vi "Shooter Controller.vi"(8 "error in":errorcluster) -> ()   [LabVIEW 2019]
doc: "This VI executes continuously carrying out the current operation and responding to updates or new operations. It will often contain the timing or control code that is difficult to place directly in TeleOp. This VI generally opens all sensors and motors and isolates the rest of the robot code from knowing how the operations are carried out."
uses:
  <vilib>/Rock Robotics/WPI/Framework/Completion Status.ctl
  Shooter Setpoints.ctl
  Shooter Operations.ctl
  <vilib>/Rock Robotics/WPI/ThirdParty/REV Robotics/SPARK MAX/Typedef/Spark MAX Idle Mode.ctl
  <vilib>/Rock Robotics/WPI/ThirdParty/REV Robotics/SPARK MAX/Typedef/Spark MAX Control Type.ctl
  <vilib>/Rock Robotics/Network Tables/NT Read Boolean.vi
  Framework/Robot Global Data.vi
  <vilib>/Rock Robotics/Network Tables/NT Read Number.vi
  <vilib>/Rock Robotics/Network Tables/NT Write Number.vi
  <vilib>/Rock Robotics/Network Tables/NT Write Boolean.vi
panel:
  out "Waveform Chart 2":dbl(graph)
  out "Waveform Chart":dbl(graph)
  in  "Interactive Values":T1
  out "Current\nCmd":string
  in  "Buttons":cluster{"Execute Cmd":bool, "Abort Cmd":bool}
  out "Command Timing":cluster{"Start Time (ms)":u32, "Iterations":i32}
  out "Status":T3
  # "Tip: It may be helpful to observe inputs and sensor values.\nYou may also want to display tuning or debugging controls."
  # "80 amps, old PID"
  # "Interactive Command: You may fill in the settings for a command\nand schedule it with the Execute button. You can observe and abort\nany command while fine tuning the code for the controller."
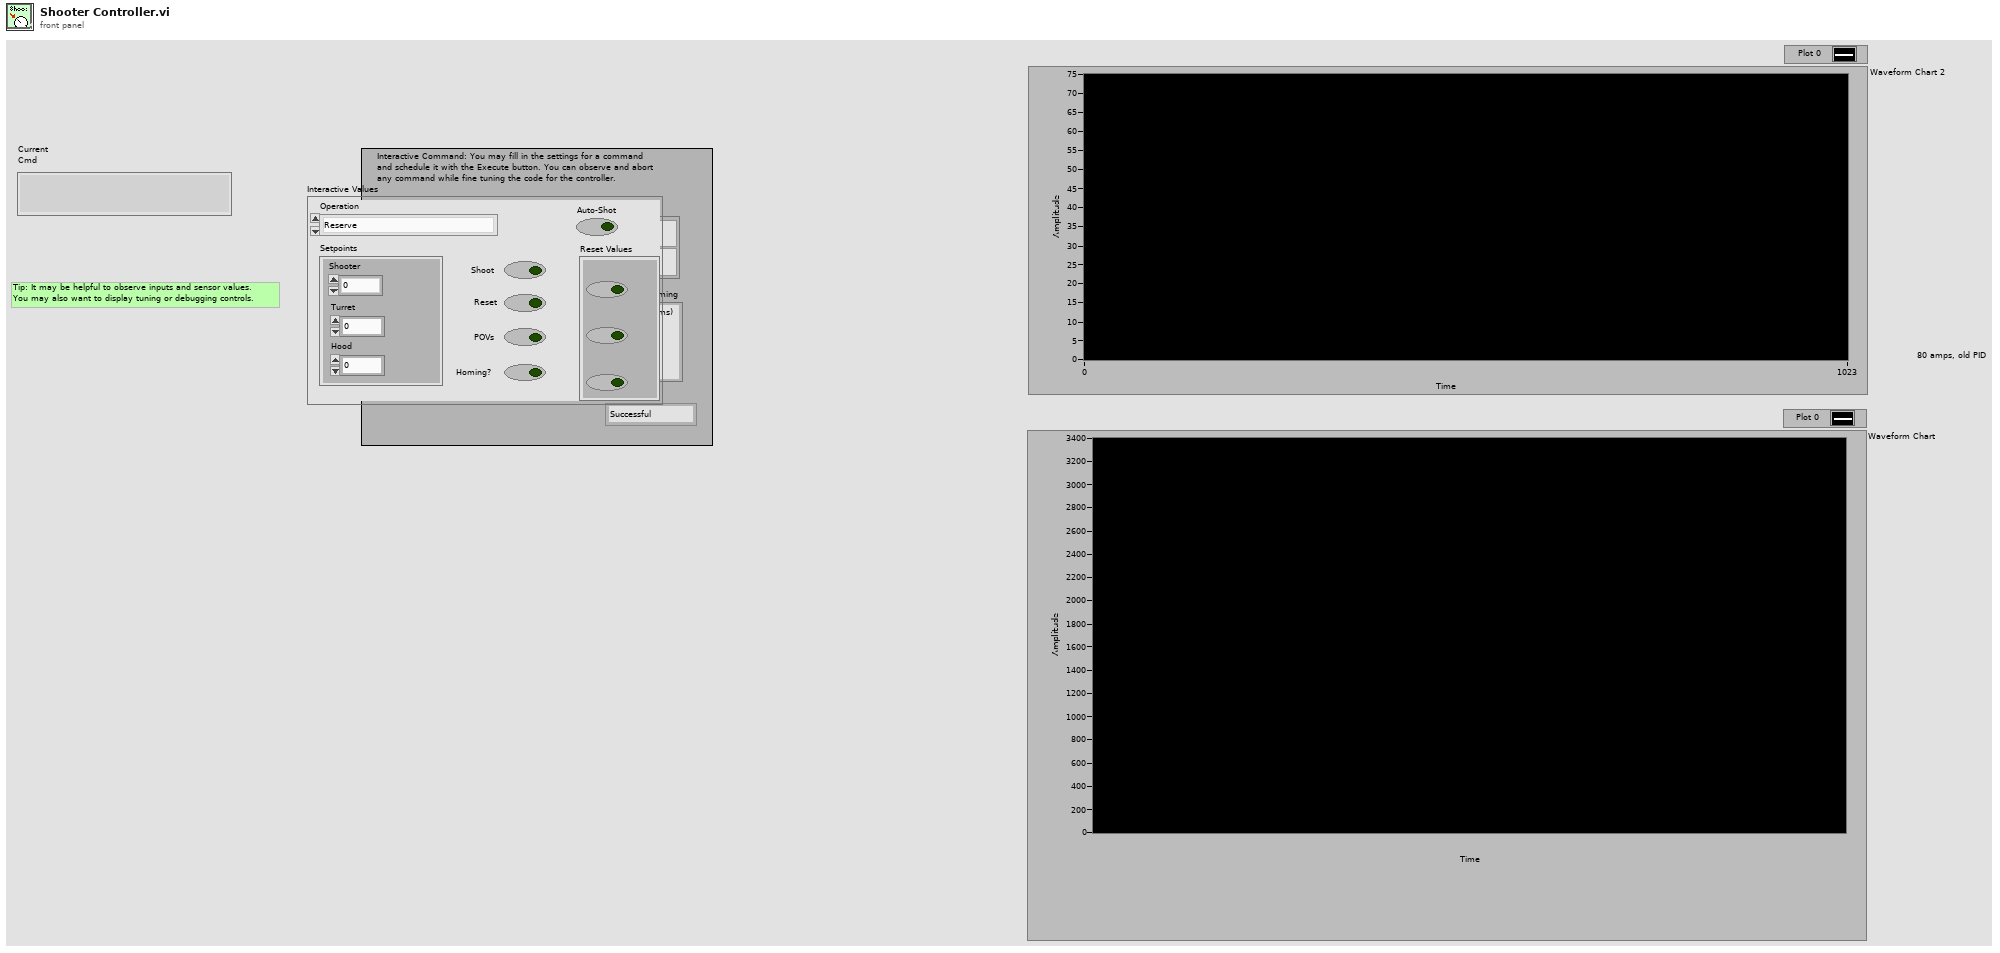
[diagram p1: front panel]
types:
  T1 = typedef "Shooter Setpoints.ctl" = cluster{"Operation":T2, "Setpoints":cluster{"Shooter":dbl, "Turret":dbl, "Hood":dbl}, "Reset Values":cluster{"Shooter Reset":bool, "Turret Reset":bool, "Hood Reset":bool}, "Auto-Shot":bool, "Shoot":bool, "Reset":bool, "POVs":bool, "Homing?":bool}
  T2 = typedef "Shooter Operations.ctl" = enum16{"Reserve", "Read Current", "Immediate"}
  T3 = typedef "Completion Status.ctl" = enum16{"Successful", "Aborted", "Incomplete"}
  T4 = cluster{"P Gain":dbl, "I Gain":dbl, "D Gain":dbl, "F Gain":dbl, "I Zone":dbl, "Min Output":dbl, "Max Output":dbl}
  T5 = typedef "Spark MAX Idle Mode.ctl" = enum16{"Coast", "Brake"}
  T6 = typedef "WPI_MotorControlDeviceRef.ctl" = cluster{"DeviceStatus":errorcluster, "Type":T7, "PWM":cluster{"PWM Channel":T8, "DeadBand":T9}, "CAN":cluster{"Device Number":u8, "SetOutput VI Ref":variant, "GetOutput VI Ref":variant, "Enable VI Ref":variant, "Disable VI Ref":variant, "Data":variant}, "Invert":bool, "DIO PWM":cluster{"PWM \"Enable\" Channel":T8, "DIOChannel":T10, "PWM Rate":dbl}}
  T7 = typedef "WPI_MotorControlType.ctl" = enum16{"PWM", "CAN", "DIO PWM"}
  T8 = typedef "FPGA_DIOPWMChannel.ctl" = enum8{"PWM 0", "PWM 1", "PWM 2", "PWM 3", "PWM 4", "PWM 5", "PWM 6", "PWM 7", "PWM 8", "PWM 9", "PWM MXP 0", "PWM MXP 1", "PWM MXP 2", "PWM MXP 3", "PWM MXP 4", "PWM MXP 5", "PWM MXP 6", "PWM MXP 7", "PWM MXP 8", "PWM MXP 9", "Invalid"}
  T9 = typedef "WPI_PWMDeadband.ctl" = cluster{"Name":string, "maxPositivePwm":i32, "minPositivePwm":i32, "centerPwm":i32, "maxNegativePwm":i32, "minNegativePwm":i32, "angularRange":u16}
  T10 = typedef "FPGA_DIOChannel.ctl" = enum8{"DIO 0", "DIO 1", "DIO 2", "DIO 3", "DIO 4", "DIO 5", "DIO 6", "DIO 7", "DIO 8", "DIO 9", "DIO MXP 0", "DIO MXP 1", "DIO MXP 2", "DIO MXP 3", "DIO MXP 4", "DIO MXP 5", "DIO MXP 6", "DIO MXP 7", "DIO MXP 8", "DIO MXP 9", "DIO MXP 10", "DIO MXP 11", "DIO MXP 12", "DIO MXP 13", "DIO MXP 14", "DIO MXP 15", "SPI Port CS1", "SPI Port CS2", "SPI Port CS3", "SPI Port MISO", "SPI Port MOSI", "Invalid"}
  T11 = typedef "Command Status Info.ctl" = cluster{"Name":string, "Status":T3, "notifier out":T12}
  T12 = typedef "Completion Notifier.ctl" = refnum<notifier>
  T13 = cluster{"Current Command":T1, "Command Timing":cluster{"Start Time (ms)":u32, "Iterations":i32}, "Command Arguments":cluster{"Command Info":T11, "Description":string, "Default Command":T1, "queue out":refnum<queue>, "Subsystem Name":string}}
  T14 = typedef "ADIS16448 Device Reference.ctl" = cluster{"DevStatus":errorcluster, "Hardware Config":T15, "Calibration Complete":refnum<notifier>, "Last Value Reference":refnum<data-value>, "Sychronous Process VI":T18, "Cmd FIFO":refnum<k33>, "Source":T19, "IMU Status LED Pin":T10, "Calibration Time":u32}
  T15 = typedef "ADIS16448 Hardware Configuration.ctl" = cluster{"SPI Clock Rate (Hz)":dbl, "IMU SPI Mode (3)":T16, "IMU Reset Pin":T10, "IMU SPI Bus":T17, "IMU Data Ready Pin":T10, "Stall Config":cluster{"Pow2BytesPerRead":u8, "StallTicks":u16, "CsToSclkTicks":u8}, "IMU Status LED Pin":T10}
  T16 = typedef "WPI_SPIMode.ctl" = enum16{"Mode 0 (Clk Idle Low,Sample on Leading)", "Mode 1 (Clk Idle Low,Sample on Trailing)", "Mode 2 (Clk Idle High,Sample on Leading)", "Mode 3 (Clk Idle High,Sample on Trailing)"}
  T17 = typedef "spi_bus.ctl" = enum16{"SPI On-Board, CS0", "SPI On-Board, CS1", "SPI On-Board, CS2", "SPI On-Board, CS3", "SPI MXP", "Invalid"}
  T18 = typedef "ADIS16448 Process.ctl" = refnum<vi>
  T19 = typedef "FPGA_CounterEncoderSourceConvertionLVSourceType.ctl" = cluster{"DevStatus":errorcluster, "AnalogTriggerMode?":bool, "DigitalMode":cluster{"DIO Channel":T20}, "AnalogTriggerMode":cluster{"AnalogTriggerIndex":T21, "OutputType":T22}}
  T20 = typedef "FPGA_DIODigitalSourceChannel.ctl" = enum8{"DIO 0", "DIO 1", "DIO 2", "DIO 3", "DIO 4", "DIO 5", "DIO 6", "DIO 7", "DIO 8", "DIO 9", "DIO MXP 0", "DIO MXP 1", "DIO MXP 2", "DIO MXP 3", "DIO MXP 4", "DIO MXP 5", "DIO MXP 6", "DIO MXP 7", "DIO MXP 8", "DIO MXP 9", "DIO MXP 10", "DIO MXP 11", "DIO MXP 12", "DIO MXP 13", "DIO MXP 14", "DIO MXP 15", "SPI Port CS1", "SPI Port CS2", "SPI Port CS3", "SPI Port MISO", "SPI Port MOSI", "Disabled"}
  T21 = typedef "FPGA_AnalogTriggerIndex.ctl" = enum8{"Trig 0", "Trig 1", "Trig 2", "Trig 3", "Trig 4", "Trig 5", "Trig 6", "Trig 7", "Invalid"}
  T22 = typedef "FPGA_AnalogTriggerOutType.ctl" = enum16{"InWindow", "TriggerState", "Rising", "Falling"}
  T23 = typedef "Spark MAX Control Type.ctl" = enum16{"Percent VBus", "Voltage", "Velocity", "Position", "Smart Motion", "Current", "Smart Velocity"}
  T24 = cluster{"Shooter Reset":bool, "Turret Reset":bool, "Hood Reset":bool}
  T25 = typedef "ADIS16448 Data.ctl" = cluster{"XAngle":dbl, "YAngle":dbl, "ZAngle":dbl}
  T26 = cluster{u32, "Setpoints":cluster{"Shooter":dbl, "Turret":dbl, "Hood":dbl}}
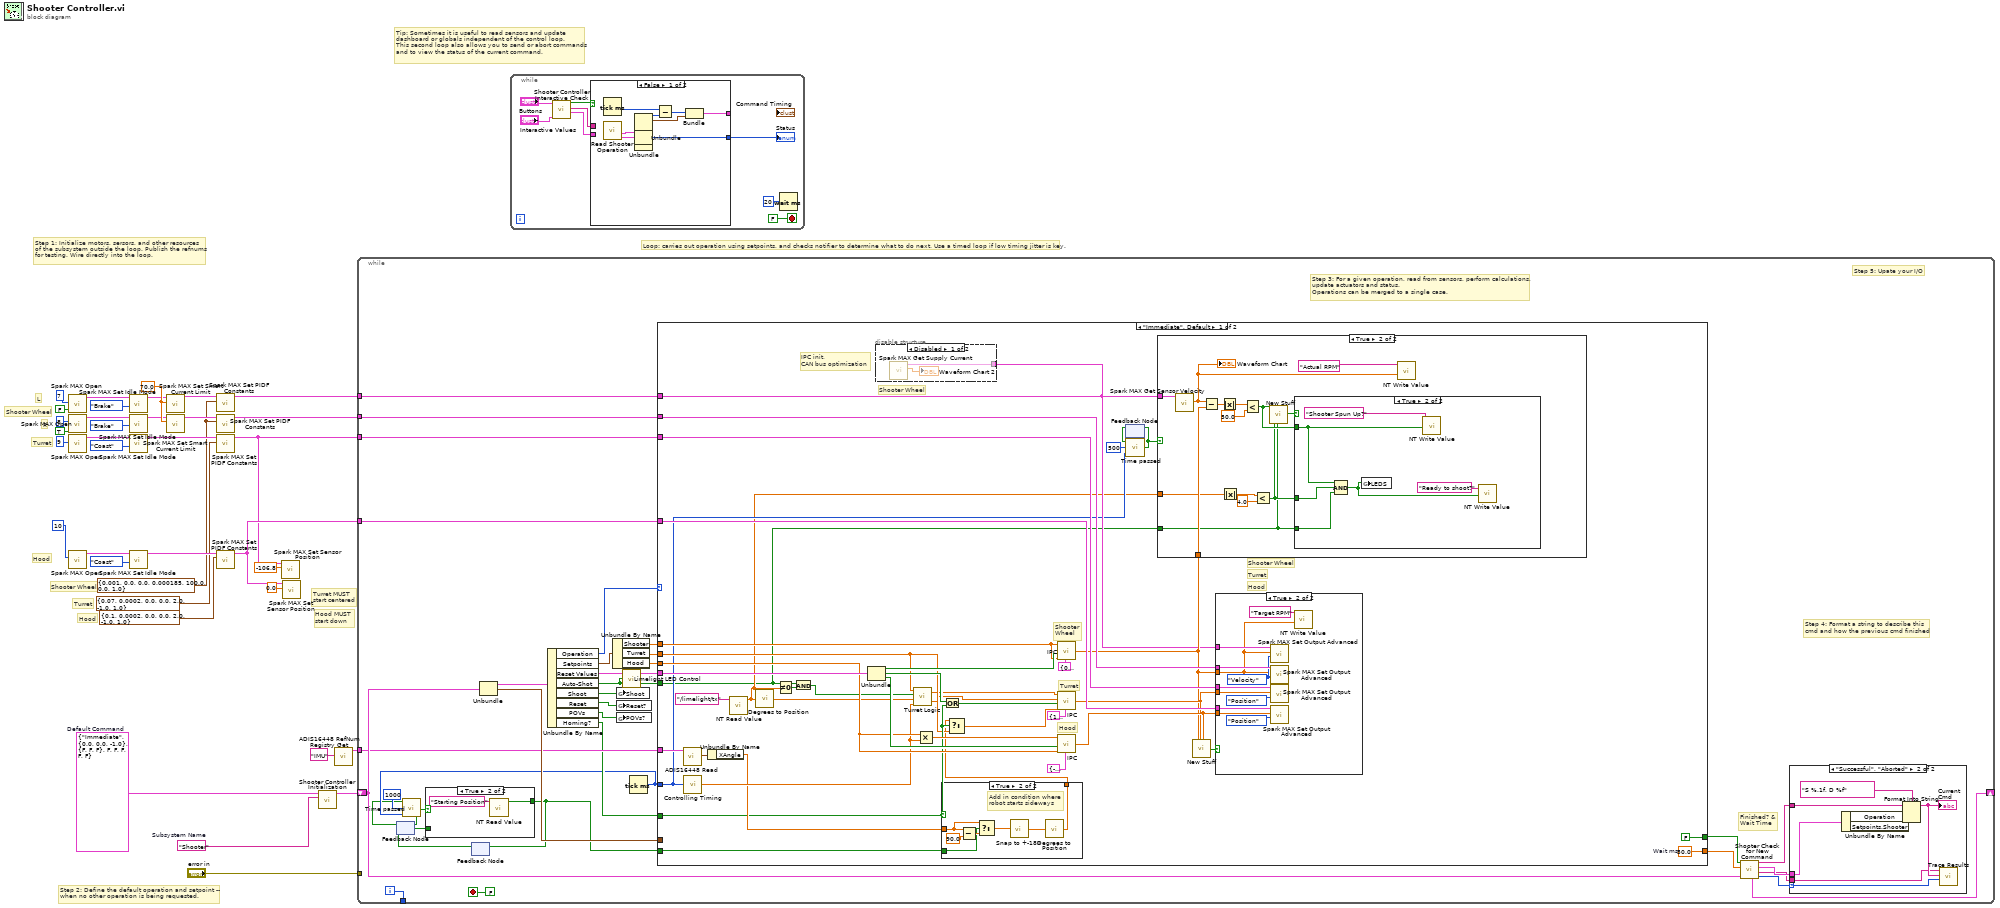
[diagram p0: block diagram]
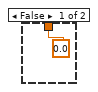
[diagram p6: hidden frame]
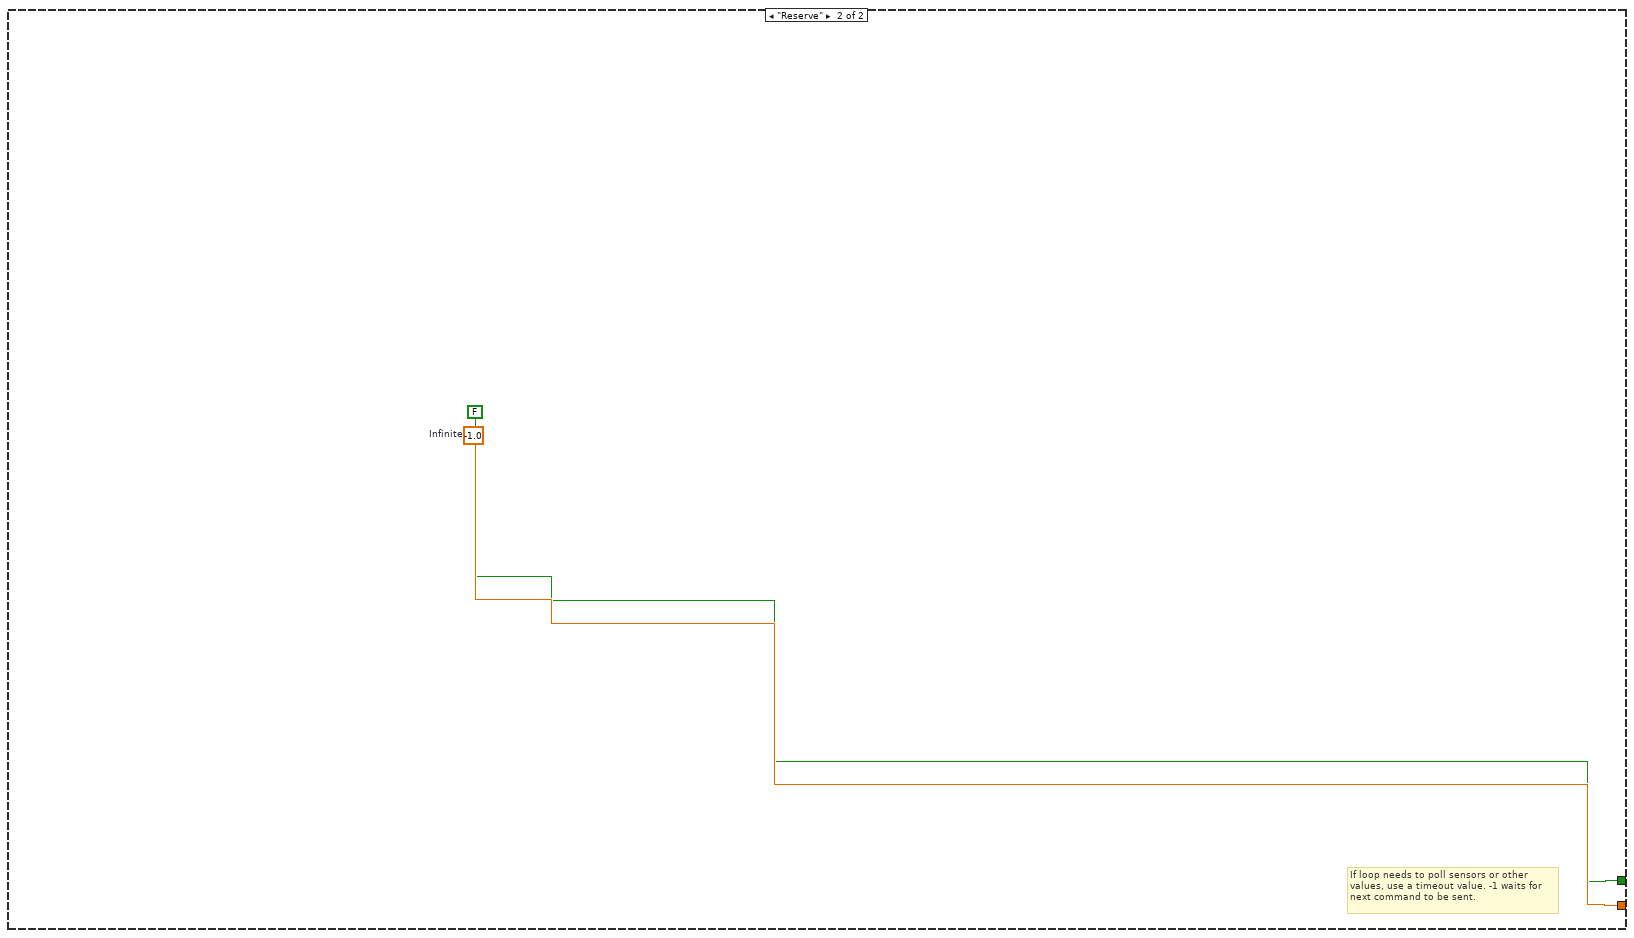
[diagram p8: hidden frame]
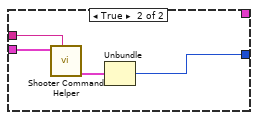
[diagram p10: hidden frame]
diagram:
  w6 = T4 {"P Gain"=0.001, "I Gain"=0.0, "D Gain"=0.0, "F Gain"=0.000185, "I Zone"=100.0, "Min Output"=0.0, "Max Output"=1.0} ("Flywheel PID")
  w26 = 70.0 ("Primay Current Limit (80A)")
  w5 = T1 {"Operation"=enum."Immediate", "Setpoints"={"Shooter"=0.0, "Turret"=0.0, "Hood"=-1.0}, "Reset Values"={"Shooter Reset"=FALSE, "Turret Reset"=FALSE, "Hood Reset"=FALSE}, "Auto-Shot"=FALSE, "Shoot"=FALSE, "Reset"=FALSE, "POVs"=FALSE, "Homing?"=FALSE}  # Default Command
  w34 = "Shooter"  # Subsystem Name
  # "Hood"
  # "Turret"
  # "Shooter Wheel"
  # "R"
  # "L"
  # "Hood MUST\nstart down"
  # "Turret MUST\nstart centered"
  # "Hood"
  # "Turret"
  # "Shooter Wheel"
  # "Tip: Sometimes it is useful to read sensors and update\ndashboard or globals independent of the control loop.\nThis second loop also allows you to send or abort commands\nand to view the status of the current command."
  # "Step 2: Define the default operation and setpoint --\nwhen no other operation is being requested."
  # "Step 1: Initialize motors, sersors, and other resources\nof the subsystem outside the loop. Publish the refnums\nfor testing. Wire directly into the loop."
  # "Loop: carries out operation using setpoints, and checks notifier to determine what to do next. Use a timed loop if low timing jitter is key."
  n1 = call <vilib>:"Spark MAX Open.vi"("Invert"=FALSE, "Device Number"=u8 7) -> ("MotorControlDeviceRef"=w9:T6)  [unwired: 8 in, 1 out]
  n2 = call <vilib>:"Spark MAX Open.vi"("Invert"=TRUE, "Device Number"=u8 8) -> ("MotorControlDeviceRef"=w10:T6)  [unwired: 8 in, 1 out]
  n3 = call <vilib>:"Spark MAX Open.vi"("Device Number"=u8 9) -> ("MotorControlDeviceRef"=w22:T6)  [unwired: 9 in, 1 out]
  n4 = call <vilib>:"Spark MAX Open.vi"("Device Number"=u8 10) -> ("MotorControlDeviceRef"=w21:T6)  [unwired: 9 in, 1 out]
  n5 = call <vilib>:"Spark MAX Set Idle Mode.vi"("Idle Mode"=Spark_MAX_Idle_Mode."Brake", "MotorControlDeviceRef in"=w9) -> ("MotorControlDeviceRef out"=w8:T6)  [unwired: 8 in, 1 out]
  n6 = call <vilib>:"Spark MAX Set Idle Mode.vi"("Idle Mode"=Spark_MAX_Idle_Mode."Brake", "MotorControlDeviceRef in"=w10) -> ("MotorControlDeviceRef out"=w7:T6)  [unwired: 8 in, 1 out]
  n7 = call <vilib>:"Spark MAX Set Idle Mode.vi"("Idle Mode"=Spark_MAX_Idle_Mode."Coast", "MotorControlDeviceRef in"=w22) -> ("MotorControlDeviceRef out"=w20:T6)  [unwired: 8 in, 1 out]
  n8 = call <vilib>:"Spark MAX Set Idle Mode.vi"("Idle Mode"=Spark_MAX_Idle_Mode."Coast", "MotorControlDeviceRef in"=w21) -> ("MotorControlDeviceRef out"=w19:T6)  [unwired: 8 in, 1 out]
  n9 = call <vilib>:"Spark MAX Set Smart Current Limit.vi"("Primay Current Limit (80A)"=w26, "MotorControlDeviceRef in"=w8) -> ("MotorControlDeviceRef out"=w14:T6)  [unwired: 8 in, 1 out]
  n10 = call <vilib>:"Spark MAX Set Smart Current Limit.vi"("Primay Current Limit (80A)"=w26, "MotorControlDeviceRef in"=w7) -> ("MotorControlDeviceRef out"=w15:T6)  [unwired: 8 in, 1 out]
  n11 = call <vilib>:"Spark MAX Set PIDF Constants.vi"("PID Constants"=w6, "MotorControlDeviceRef"=w14) -> ("MotorControlDeviceRef"=w13:T6)  [unwired: 8 in, 1 out]
  n12 = call <vilib>:"Spark MAX Set PIDF Constants.vi"("PID Constants"=w6, "MotorControlDeviceRef"=w15) -> ("MotorControlDeviceRef"=w16:T6)  [unwired: 8 in, 1 out]
  n13 = call <vilib>:"Spark MAX Set PIDF Constants.vi"("PID Constants"=T4 {"P Gain"=0.07, "I Gain"=0.0002, "D Gain"=0.0, "F Gain"=0.0, "I Zone"=2.0, "Min Output"=-1.0, "Max Output"=1.0} ("Turret PID"), "MotorControlDeviceRef"=w20) -> ("MotorControlDeviceRef"=w2:T6)  [unwired: 8 in, 1 out]
  n14 = call <vilib>:"Spark MAX Set PIDF Constants.vi"("PID Constants"=T4 {"P Gain"=0.1, "I Gain"=0.0002, "D Gain"=0.0, "F Gain"=0.0, "I Zone"=2.0, "Min Output"=-1.0, "Max Output"=1.0} ("Hood PID"), "MotorControlDeviceRef"=w19) -> ("MotorControlDeviceRef"=w4:T6)  [unwired: 8 in, 1 out]
  n15 = call <vilib>:"Spark MAX Set Sensor Position.vi"("Position"=-106.8, "MotorControlDeviceRef"=w2) -> ()  [unwired: 8 in, 2 out]
  n16 = call <vilib>:"Spark MAX Set Sensor Position.vi"("Position"=0.0, "MotorControlDeviceRef"=w4) -> ()  [unwired: 8 in, 2 out]
  n17 = call "Shooter Controller Initialization.vi"("Subsystem Name"=w34, "Default Command"=w5) -> ("Current Command"=w35:T13)  [unwired: 9 in]
  n18 = call "ADIS16448 RefNum Registry Get.vi"("refnum name"="IMU") -> ("ADIS16448DevRef Out"=w28:T14)  [unwired: 9 in, 1 out]
  n19 = while {
    shift-right: [w66] -> _
    shift-left: w35 -> [w59]
    tunnel: [w69] -> _
    tunnel: "error in" -> [_]
    tunnel: w16 -> [w58]
    tunnel: w2 -> [w53]
    tunnel: w4 -> [w57]
    tunnel: w28 -> [w56]
    tunnel: w13 -> [w55]
    i -> [w69]
    stop <- FALSE stop-if-true
    # "Step 5: Upate your I/O"
    # "Step 4: Format a string to describe this\ncmd and how the previous cmd finished"
    # "Finished? &\nWait Time"
    # "Step 3: For a given operation, read from sensors, perform calculations,\nupdate actuators and status.\nOperations can be merged to a single case."
    n20 = feedback #1() -> (w39:bool)  [unwired: 1 in]
    n21 = feedback #2() -> (w40:bool)  [unwired: 1 in]
    n22 = Unbundle(w59) -> ("Current Command"=w68:T1, "Command Timing"=w67:cluster{"Start Time (ms)":u32, "Iterations":i32})  [unwired: 1 out]
    n23 = Unbundle By Name(w68) -> ("Operation"=w37:T2, "Setpoints"=w52:cluster{"Shooter":dbl, "Turret":dbl, "Hood":dbl}, "Reset Values"=w54:T24, "Auto-Shot"=w47:bool, "Shoot"=w46:bool, "Reset"=w48:bool, "POVs"=w45:bool, "Homing?"=w44:bool)
    n24 = Unbundle By Name(w52) -> ("Shooter"=w51:dbl, "Turret"=w50:dbl, "Hood"=w49:dbl)
    n25 = global write "Robot Global Data.vi" "Shoot"(w46) -> ()
    n26 = global write "Robot Global Data.vi" "Reset?"(w48) -> ()
    n27 = global write "Robot Global Data.vi" "POVs?"(w45) -> ()
    n28 = call "Limelight LED Control.vi"("Auto-Align"=w47) -> ()
    n29 = Tick Count (ms)() -> (millisecond timer value=w41:u32)
    n30 = call "Time passed.vi"("ms timer value"=w41, "Wait time"=u32 1000 ("Time (ms)"), "Reset"=w39) -> ("Boolean out"=w38:bool)
    n31 = feedback-in #1(w38) -> ()
    n32 = case shown="True" w38 {
      tunnel: [w71 w73] -> w43
      tunnel: w40 -> [w71 _]
      frame False {
      }
      frame True {
        n33 = call-poly <vilib>:"NT Read Value.vi"("Name"="Starting Position") -> ("Boolean"=w73:bool)  [unwired: 9 in, 1 out]
      }
    }
    n34 = feedback-in #2(w43) -> ()
    n35 = case shown="\"Immediate\", Default" w37 {
      tunnel: [w115 w158] -> w64
      tunnel: [FALSE ("ignore previous (F)") FALSE ("ignore previous (F)")] -> w65
      tunnel: w67 -> [_ _]
      tunnel: w41 -> [w79 _]
      tunnel: w58 -> [w109 _]
      tunnel: w57 -> [w108 _]
      tunnel: w53 -> [w106 _]
      tunnel: w56 -> [w92 _]
      tunnel: w55 -> [w89 _]
      tunnel: w51 -> [w102 _]
      tunnel: w50 -> [w85 _]
      tunnel: w49 -> [w101 _]
      tunnel: w54 -> [w110 _]
      tunnel: w47 -> [w74 _]
      tunnel: w44 -> [w86 _]
      tunnel: w43 -> [w80 _]
      frame "Immediate", Default {
        w115 = 50.0  # Wait ms
        # "Hood"
        # "Turret"
        # "Shooter \nWheel"
        # "Hood"
        # "Turret"
        # "Shooter Wheel"
        # "Shooter Wheel"
        # "IPC init,\nCAN bus optimization"
        n36 = call "ADIS16448 Read.vi"("ADIS16448DevRef"=w92) -> ("Gyro Value"=w91:T25)  [unwired: 3 in, 7 out]
        n37 = call "Controlling Timing.vi"("Time"=w79) -> ("New Time"=w94:dbl)
        n38 = Unbundle By Name(w91) -> ("XAngle"=w90:dbl)
        n39 = call-poly <vilib>:"NT Read Value.vi"("Name"="/limelight/tx") -> ("Numeric"=w75:dbl)  [unwired: 9 in, 1 out]
        n40 = call "Degrees to Position.vi"("Degree"=w75) -> ("Encoder Position"=w95:dbl)  [unwired: 4 in]
        n41 = Not Equal To 0?(x=w75) -> (x != 0?=w100:bool)
        n42 = And(x=w74, y=w100) -> (x .and. y?=w96:bool)
        n43 = Unbundle(w110) -> ("Shooter Reset"=w103:bool, "Turret Reset"=w88:bool, "Hood Reset"=w104:bool)
        n44 = disable-structure shown="Disabled" {
          disable-tunnel: w89 -> [w137 _]
          frame Disabled {
            n45 = call <vilib>:"Spark MAX Get Supply Current.vi"("MotorControlDevRef in"=w137) -> ("Current"=→"Waveform Chart 2":dbl)  [unwired: 7 in, 3 out]
          }
          frame Enabled {
          }
        }
        n46 = call "Turret Logic.vi"("Turret Input"=w85, "Turn Turret?"=w96, "Ticks"=w95, "Timing"=w94) -> ("Value"=w81:dbl, "Multiplier"=w82:dbl)  [unwired: 1 in]
        n47 = Multiply(x=w101, y=w94) -> (x*y=w111:dbl)
        n48 = case shown="True" w86 {
          tunnel: w90 -> [_ w142]
          tunnel: [0.0 ("Encoder Position") w144] -> w84
          tunnel: w80 -> [_ w139]
          frame False {
          }
          frame True {
            # "Add in condition where \nrobot starts sideways"
            n49 = Subtract(x=w142, y=90.0) -> (x-y=w141:dbl)
            n50 = Select(t=w142, s=w139, f=w141) -> (s? t:f=w143:dbl)
            n51 = call "Snap to +-180.vi"("Slide"=w143) -> ("Slide 2"=w145:dbl)
            n52 = call "Degrees to Position.vi"("Degree"=w145) -> ("Encoder Position"=w144:dbl)  [unwired: 4 in]
          }
        }
        n53 = Or(x=w88, y=w86) -> (x .or. y?=w87:bool)
        n54 = Select(t=w84, s=w86, f=w85) -> (s? t:f=w83:dbl)
        n55 = call "IPC.vi"("Coerced Values"=cluster{"Max":dbl, "Min":dbl, "Coerce?":bool} {"Max"=0.0, "Min"=0.0, "Coerce?"=FALSE}, "Initilization"=w102, "Reset"=w103, "Value"=w102) -> ("IPCed"=w93:dbl)  [unwired: 2 in]
        n56 = call "IPC.vi"("Coerced Values"=cluster{"Max":dbl, "Min":dbl, "Coerce?":bool} {"Max"=106.8, "Min"=-106.8, "Coerce?"=TRUE}, "Initilization"=w83, "Reset"=w87, "Multiplier"=w82, "Value"=w81) -> ("IPCed"=w105:dbl)  [unwired: 1 in]
        n57 = call "IPC.vi"("Coerced Values"=cluster{"Max":dbl, "Min":dbl, "Coerce?":bool} {"Max"=-0.5, "Min"=-17.0, "Coerce?"=TRUE}, "Initilization"=w101, "Reset"=w104, "Value"=w111) -> ("IPCed"=w112:dbl)  [unwired: 2 in]
        n58 = feedback #3() -> (w78:bool)  [unwired: 1 in]
        n59 = call "Time passed.vi"("ms timer value"=w79, "Wait time"=u32 500, "Reset"=w78) -> ("Boolean out"=w76:bool)
        n60 = feedback-in #3(w76) -> ()
        n61 = case shown="True" w76 {
          tunnel: w93 -> [_ w123]
          tunnel: w89 -> [_ w121]
          tunnel: w75 -> [_ w120]
          tunnel: w74 -> [_ w116]
          frame False {
          }
          frame True {
            n62 = call <vilib>:"Spark MAX Get Sensor Velocity.vi"("MotorControlDevRef in"=w121) -> ("Sensor Velocity"=w122:dbl)  [unwired: 7 in, 3 out]
            "Waveform Chart" <- w122
            n63 = Subtract(x=w122, y=w123) -> (x-y=w129:dbl)
            n64 = Absolute Value(x=w129) -> (abs(x)=w128:dbl)
            n65 = Absolute Value(x=w120) -> (abs(x)=w119:dbl)
            n66 = Less?(x=w128, y=50.0) -> (x < y?=w125:bool)
            n67 = Less?(x=w119, y=4.0) -> (x < y?=w117:bool)
            n68 = call "New Stuff.vi"("Variant"=w125, "Variant 13"=w117, "Variant 6"=w116) -> ("x != y?"=w126:bool)  [unwired: 24 in]
            n69 = case shown="True" w126 {
              tunnel: w125 -> [_ w133]
              tunnel: w117 -> [_ w132]
              tunnel: w116 -> [_ w130]
              frame False {
              }
              frame True {
                n70 = Compound Arithmetic op=AND(w133, w132, w130) -> (w131:bool)
                n71 = global write "Robot Global Data.vi" "LEDS"(w131) -> ()
                n72 = call-poly <vilib>:"NT Write Value.vi"("Boolean"=w133, "Name"="Shooter Spun Up?") -> ()  [unwired: 9 in, 1 out]
                n73 = call-poly <vilib>:"NT Write Value.vi"("Boolean"=w131, "Name"="Ready to shoot?") -> ()  [unwired: 9 in, 1 out]
              }
            }
            n74 = call-poly <vilib>:"NT Write Value.vi"("Numeric"=w122, "Name"="Actual RPM") -> ()  [unwired: 9 in, 1 out]
          }
        }
        n75 = call "New Stuff.vi"("Variant 12"=w93, "Variant 11"=w105, "Variant 10"=w112) -> ("x != y?"=w113:bool)  [unwired: 24 in]
        n76 = case shown="True" w113 {
          tunnel: w108 -> [_ w156]
          tunnel: w106 -> [_ w155]
          tunnel: w109 -> [_ w154]
          tunnel: w112 -> [_ w151]
          tunnel: w105 -> [_ w150]
          tunnel: w93 -> [_ w147]
          tunnel: w89 -> [_ w148]
          frame False {
          }
          frame True {
            w149 = Spark_MAX_Control_Type."Velocity" ("Control Mode")
            n77 = call <vilib>:"Spark MAX Set Output Advanced.vi"("Control Mode"=w149, "Setpoint"=w147, "MotorControlDevRef"=w148) -> ()  [unwired: 7 in, 2 out]
            n78 = call <vilib>:"Spark MAX Set Output Advanced.vi"("Control Mode"=w149, "Setpoint"=w147, "MotorControlDevRef"=w154) -> ()  [unwired: 7 in, 2 out]
            n79 = call <vilib>:"Spark MAX Set Output Advanced.vi"("Control Mode"=Spark_MAX_Control_Type."Position", "Setpoint"=w150, "MotorControlDevRef"=w155) -> ()  [unwired: 7 in, 2 out]
            n80 = call <vilib>:"Spark MAX Set Output Advanced.vi"("Control Mode"=Spark_MAX_Control_Type."Position", "Setpoint"=w151, "MotorControlDevRef"=w156) -> ()  [unwired: 7 in, 2 out]
            n81 = call-poly <vilib>:"NT Write Value.vi"("Numeric"=w147, "Name"="Target RPM") -> ()  [unwired: 9 in, 1 out]
          }
        }
      }
      frame "Reserve" {
        w158 = -1.0  # Infinite
        # "If loop needs to poll sensors or other\nvalues, use a timeout value. -1 waits for\nnext command to be sent."
      }
    }
    n82 = call "Shooter Check for New Command.vi"("Current Command"=w59, "Wait time (ms)"=w64, "Finished?"=w65) -> ("Completion"=w60:T3, "Subsystem Name"=w61:string, "Current Command"=w62:T1, "Initial Trace String"=w63:string, "NextCommand"=w66:T13)  [unwired: 4 in]
    n83 = case shown="\"Successful\", \"Aborted\"" w60 {
      selector: w60 -> [_ w166]
      tunnel: w63 -> [_ w162]
      tunnel: w62 -> [_ w163]
      tunnel: w61 -> [_ w160]
      frame "Incomplete", Default {
        # "Continuing current command"
      }
      frame "Successful", "Aborted" {
        # "Report and setup for next command"
        n84 = Unbundle By Name(w163) -> ("Operation"=w165:T2, "Setpoints.Shooter"=w159:dbl)
        n85 = Format Into String(format string="S %.1f, D %f", initial string=w162, w165, w159) -> (resulting string=w161:string)  [unwired: 1 in, 1 out]
        "Current\nCmd" <- w161
        n86 = call <vilib>:"Trace Results.vi"("Status of previous command"=w166, "Description"=w161, "Subsystem"=w160) -> ()  [unwired: 9 in]
      }
    }
  }
  n87 = while {
    stop <- FALSE stop-if-true
    n88 = call "Shooter Controller Interactive Check.vi"("Interactive Command in"="Interactive Values", "Buttons"="Buttons") -> ("Interactive Command out"=w169:T1, "Trace String"=w170:string, "Schedule"=w171:bool)  [unwired: 7 in]
    n89 = case shown="False" w171 {
      tunnel: [w182 w186] -> w168
      tunnel: w169 -> [_ w184]
      tunnel: [w178 _] -> _
      tunnel: w170 -> [_ w185]
      frame False {
        n90 = Tick Count (ms)() -> (millisecond timer value=w177:u32)
        n91 = call "Read Shooter Operation.vi"() -> ("Command Info"=w175:T11, "SubSystem Data"=w176:T1)  [unwired: 9 in, 1 out]
        n92 = Unbundle(w176) -> ("Operation"=w181:T2, "Setpoints"=w179:cluster{"Shooter":dbl, "Turret":dbl, "Hood":dbl})  [unwired: 6 out]
        n93 = Unbundle(w175) -> ("Status"=w182:T3)  [unwired: 2 out]
        n94 = Subtract(x=w177, y=w181) -> (x-y=w180:u32)
        n95 = Bundle(w180, "Setpoints"=w179) -> (w178:T26)  [unwired: 1 in]
      }
      frame True {
        n96 = call "Shooter Command Helper.vi"("Description"=w185, "SubSystem Data"=w184) -> ("Command Info Out"=w183:T11)  [unwired: 7 in, 2 out]
        n97 = Unbundle(w183) -> ("Status"=w186:T3)  [unwired: 2 out]
      }
    }
    "Status" <- w168
    n98 = Wait (ms)(milliseconds to wait=u32 20) -> ()  [unwired: 1 out]
  }
